vi "Exec2017.vi"(8 "Commands in":string) -> (3 "Commands out":string, 4 "File not found or missing parameters":bool)   [LabVIEW 2017]
uses:
  <vilib>/regexp/Match Regular Expression.xnode
panel:
  out "File not found":bool
  out "Program Finished":bool
  out "Missing parameters":bool
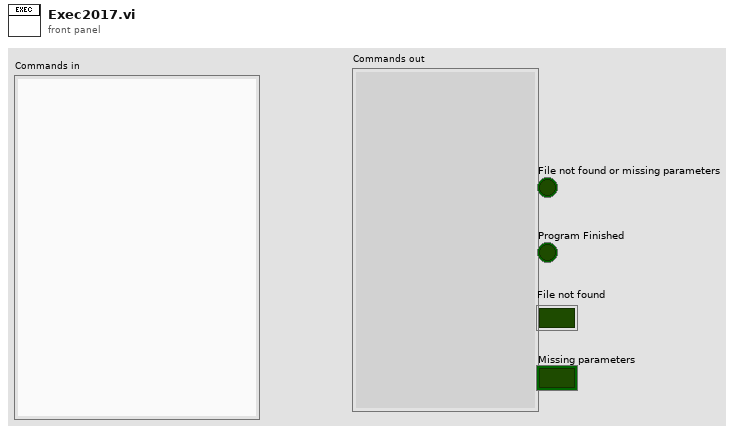
[diagram p1: front panel]
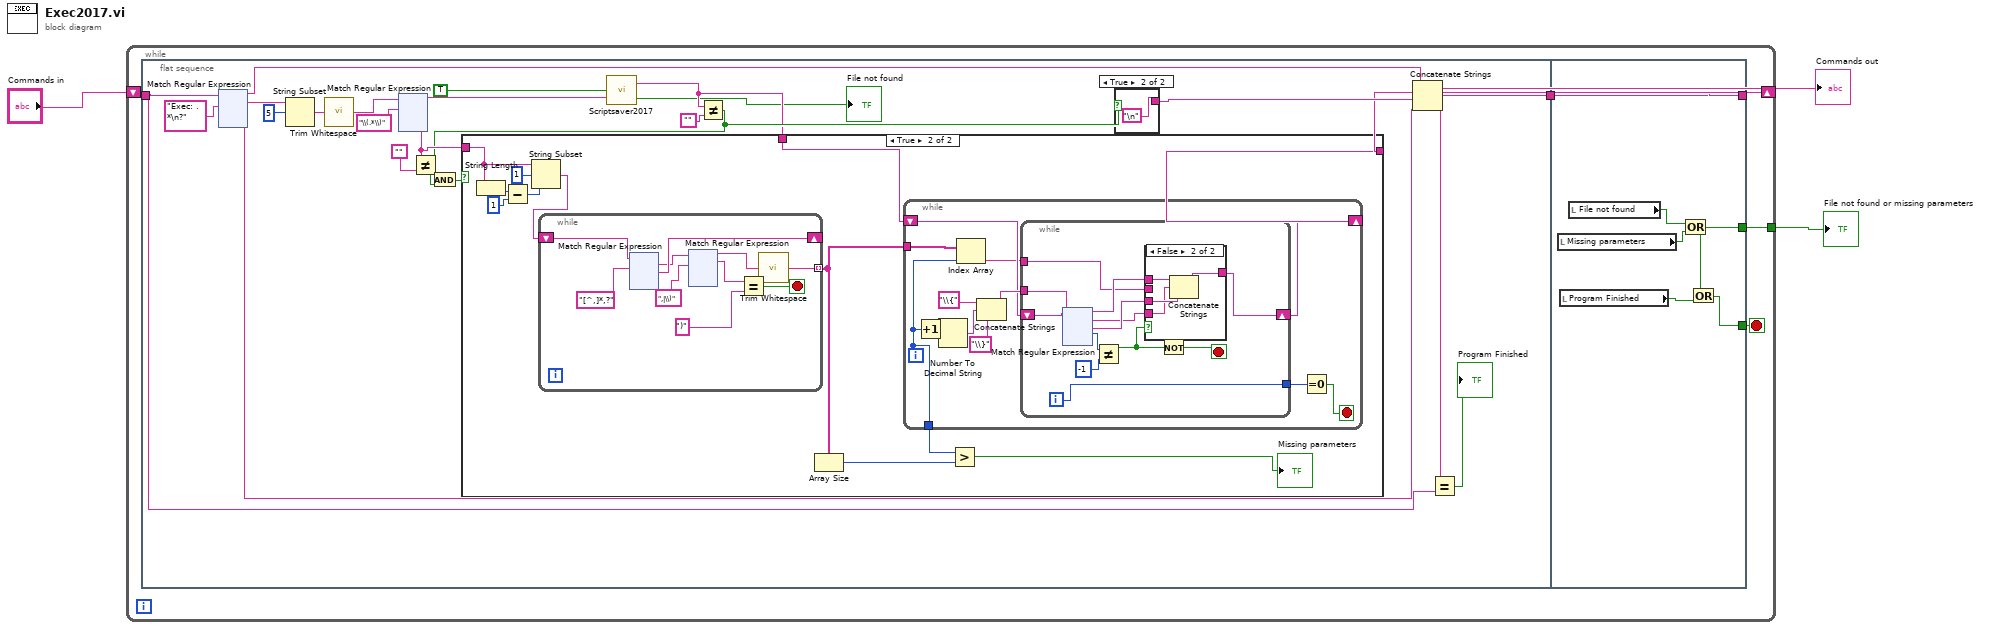
[diagram p0: block diagram]
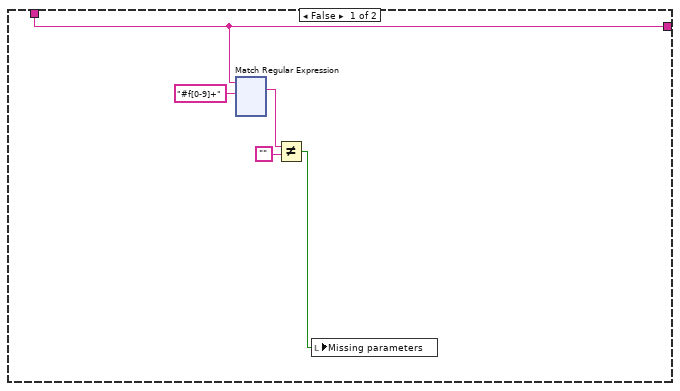
[diagram p2: hidden frame]
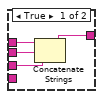
[diagram p3: hidden frame]
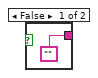
[diagram p4: hidden frame]
diagram:
  n1 = while {
    shift-right: [w8] -> w2
    shift-left: "Commands in" -> [w7]
    tunnel: [w4] -> w1
    stop <- w5 stop-if-true
    n2 = flat-sequence {
      tunnel: w7 -> [w22]
      tunnel: [w23] -> w6
      tunnel: [w782] -> w8
      tunnel: w6 -> [w782]
      tunnel: [w778] -> w5
      tunnel: [w777] -> w4
      frame #0 {
        n3 = xnode "Match Regular Expression"("input string"=w22, "regular expression"="Exec: .*\n?") -> ("before match"=w27:string, "whole match"=w30:string, "after match"=w25:string)  [unwired: 4 in, 2 out]
        n4 = String Subset(string=w30, offset (0)=5) -> (substring=w26:string)  [unwired: 1 in]
        n5 = call <vilib>:"Trim Whitespace.vi"("string"=w26) -> ("trimmed string"=w20:string)  [unwired: 1 in]
        n6 = xnode "Match Regular Expression"("input string"=w20, "regular expression"="\\(.*\\)") -> ("before match"=w18:string, "whole match"=w16:string)  [unwired: 4 in, 3 out]
        n7 = Not Equal?(x=w16, y="") -> (x != y?=w15:bool)
        n8 = call "Scriptsaver2017.vi"("Filename"=w18, "Save (0)/Load (1)"=TRUE) -> ("File not found"=→"File not found":bool, "Loaded Script"=w12:string)  [unwired: 1 in]
        n9 = Not Equal?(x=w12, y="") -> (x != y?=w14:bool)
        n10 = And(x=w14, y=w15) -> (x .and. y?=w13:bool)
        n11 = case shown="True" w13 {
          tunnel: w16 -> [_ w156]
          tunnel: w12 -> [w35 w161]
          tunnel: [w35 w160] -> w11
          frame False {
            n12 = xnode "Match Regular Expression"("input string"=w35, "regular expression"="#f[0-9]+") -> ("whole match"=w33:string)  [unwired: 4 in, 4 out]
            n13 = Not Equal?(x=w33, y="") -> (x != y?=w32:bool)
            n14 = local write "Missing parameters"(w32) -> ()
          }
          frame True {
            n15 = String Length(string=w156) -> (length=w159:i32)
            n16 = Subtract(x=w159, y=1) -> (x-y=w157:i32)
            n17 = String Subset(string=w156, offset (0)=1, length (rest)=w157) -> (substring=w154:string)
            n18 = while {
              tunnel: [w311] -> w162 mode=indexing
              shift-right: [w316] -> _
              shift-left: w154 -> [w317]
              stop <- w314 stop-if-true
              n19 = xnode "Match Regular Expression"("input string"=w317, "regular expression"="[^,]*,?") -> ("whole match"=w312:string, "after match"=w316:string)  [unwired: 4 in, 3 out]
              n20 = xnode "Match Regular Expression"("input string"=w312, "regular expression"=",|\\)") -> ("before match"=w310:string, "whole match"=w309:string)  [unwired: 4 in, 3 out]
              n21 = Equal?(x=w309, y=")" ("String")) -> (x = y?=w314:bool)
              n22 = call <vilib>:"Trim Whitespace.vi"("string"=w310) -> ("trimmed string"=w311:string)  [unwired: 1 in]
            }
            n23 = Array Size(array=w162) -> (size(s)=w153:i32)
            n24 = while {
              tunnel: w162 -> [w168]
              shift-right: [w169] -> w160
              shift-left: w161 -> [w170]
              tunnel: [w163] -> w152
              i -> [w163]
              stop <- w165 stop-if-true
              n25 = Increment(x=w163) -> (x+1=w172:i32)
              n26 = Number To Decimal String(number=w172) -> (decimal integer string=w174:string)  [unwired: 1 in]
              n27 = Index Array(array=w168, index=w163) -> (element=w167:string)
              n28 = Concatenate Strings("\\{" ("string"), w174, "\\}" ("string")) -> (w171:string)
              n29 = while {
                tunnel: w171 -> [w186]
                tunnel: w167 -> [w178]
                shift-right: [w182] -> w169
                shift-left: w170 -> [w185]
                tunnel: [w175] -> w164
                i -> [w175]
                stop <- w177 stop-if-true
                n30 = xnode "Match Regular Expression"("input string"=w185, "regular expression"=w186) -> ("before match"=w184:string, "whole match"=w181:string, "after match"=w183:string, "offset past match"=w180:i32)  [unwired: 4 in, 1 out]
                n31 = Not Equal?(x=w180, y=-1) -> (x != y?=w176:bool)
                n32 = case shown="False" w176 {
                  tunnel: w184 -> [w190 w194]
                  tunnel: w183 -> [w189 w193]
                  tunnel: w178 -> [w188 _]
                  tunnel: [w187 w192] -> w182
                  tunnel: w181 -> [_ w191]
                  frame True {
                    n33 = Concatenate Strings(w190, w188, w189) -> (w187:string)
                  }
                  frame False {
                    n34 = Concatenate Strings(w194, w191, w193) -> (w192:string)
                  }
                }
                n35 = Not(x=w176) -> (.not. x?=w177:bool)
              }
              n36 = Equal To 0?(x=w164) -> (x = 0?=w165:bool)
            }
            n37 = Greater?(x=w152, y=w153) -> (0:→"Missing parameters":bool)
          }
        }
        n38 = case shown="True" w14 {
          tunnel: ["" "\n"] -> w24
          frame False {
          }
          frame True {
          }
        }
        n39 = Concatenate Strings(w27, w11, w24, w25) -> (w23:string)
        n40 = Equal?(x=w23, y=w22) -> (x = y?=→"Program Finished":bool)
      }
      frame #1 {
        n41 = local read "Missing parameters"() -> (w780:bool)
        n42 = local read "Program Finished"() -> (w779:bool)
        n43 = local read "File not found"() -> (w781:bool)
        n44 = Or(x=w781, y=w780) -> (x .or. y?=w777:bool)
        n45 = Or(x=w777, y=w779) -> (x .or. y?=w778:bool)
      }
    }
  }
  "Commands out" <- w2
  "File not found or missing parameters" <- w1
